vi "Test_Environment.vi"() -> ()   [LabVIEW 2016]
panel:
  out "Environment":enum16{"Matlab", "LabVIEW"}(ring)
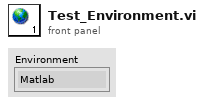
[diagram p1: front panel]
diagram:
